vi "testDataPass_v2,0_vi2.vi"() -> ()   [LabVIEW 2014]
uses:
  testDataPass_v2,0_global1.vi
panel:
  in  "stop":bool
  out "arrTF_read":bool[](array[boolean])
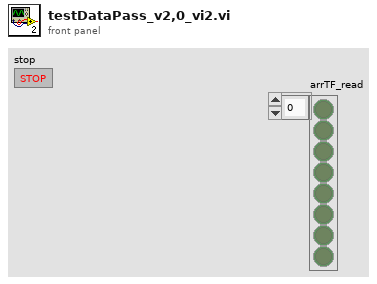
[diagram p1: front panel]
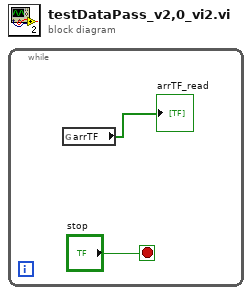
[diagram p0: block diagram]
diagram:
  n1 = while {
    stop <- "stop" stop-if-true
    n2 = global read "testDataPass_v2,0_global1.vi" "arrTF"() -> (→"arrTF_read":bool[])
  }
